vi "XYRange_Default_View.vi"(0 "SygZad Podg Ref":refnum<vi>, 1 "Radio Buttons":T1(radio), 2 "Offset ACDist":dbl, 3 "Offset":dbl, 4 "Amplituda":dbl, 5 "error in (no error)":errorcluster) -> (19 "error out":errorcluster)   [LabVIEW 2021]
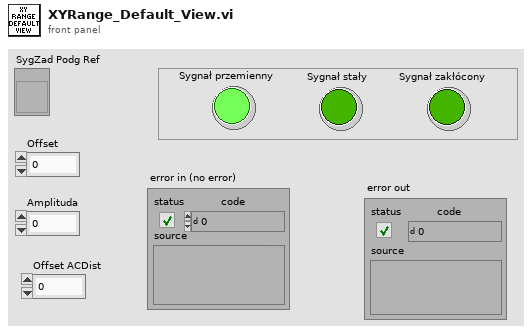
[diagram p1: front panel]
types:
  T1 = enum32{"Sygnał przemienny", "Sygnał stały", "Sygnał zakłócony"}
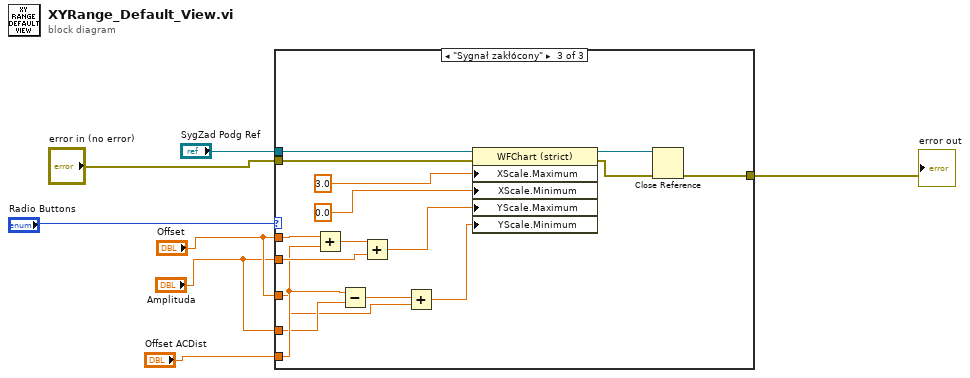
[diagram p0: block diagram]
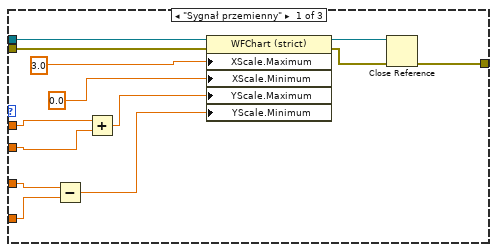
[diagram p2: hidden frame]
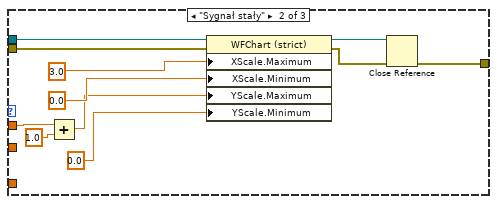
[diagram p3: hidden frame]
diagram:
  n1 = case shown="\"Sygnał zakłócony\"" "Radio Buttons" {
    tunnel: "SygZad Podg Ref" -> [w20 w31 w47]
    tunnel: "error in (no error)" -> [w18 w29 w45]
    tunnel: [w16 w27 w43] -> w5
    tunnel: "Offset" -> [w8 w24 w40]
    tunnel: "Amplituda" -> [w12 _ w38]
    tunnel: "Offset" -> [w11 _ w33]
    tunnel: "Amplituda" -> [w10 _ w35]
    tunnel: "Offset ACDist" -> [_ _ w36]
    frame "Sygnał przemienny" {
      n2 = Subtract(x=w11, y=w10) -> (x-y=w9:dbl)
      n3 = Add(x=w8, y=w12) -> (x+y=w13:dbl)
      n4 = property class="WFChart (strict)"(reference=w20, error in=w18, "XScale.Maximum"=3.0 ("X Scale.Range:Maximum"), "XScale.Minimum"=0.0 ("X Scale.Range:Minimum"), "YScale.Maximum"=w13, "YScale.Minimum"=w9) -> (reference out=w19:refnum<vi>, error out=w17:errorcluster)
      n5 = Close Reference(reference=w19, error in (no error)=w17) -> (error out=w16:errorcluster)
    }
    frame "Sygnał stały" {
      n6 = Add(x=w24, y=1.0) -> (x+y=w23:dbl)
      n7 = property class="WFChart (strict)"(reference=w31, error in=w29, "XScale.Maximum"=3.0 ("X Scale.Range:Maximum"), "XScale.Minimum"=0.0 ("X Scale.Range:Minimum"), "YScale.Maximum"=w23, "YScale.Minimum"=0.0 ("Y Scale.Range:Minimum")) -> (reference out=w30:refnum<vi>, error out=w28:errorcluster)
      n8 = Close Reference(reference=w30, error in (no error)=w28) -> (error out=w27:errorcluster)
    }
    frame "Sygnał zakłócony" {
      n9 = Add(x=w40, y=w36) -> (x+y=w39:dbl)
      n10 = Subtract(x=w36, y=w35) -> (x-y=w34:dbl)
      n11 = Add(x=w39, y=w38) -> (x+y=w37:dbl)
      n12 = Add(x=w34, y=w33) -> (x+y=w32:dbl)
      n13 = property class="WFChart (strict)"(reference=w47, error in=w45, "XScale.Maximum"=3.0 ("X Scale.Range:Maximum"), "XScale.Minimum"=0.0 ("X Scale.Range:Minimum"), "YScale.Maximum"=w37, "YScale.Minimum"=w32) -> (reference out=w46:refnum<vi>, error out=w44:errorcluster)
      n14 = Close Reference(reference=w46, error in (no error)=w44) -> (error out=w43:errorcluster)
    }
  }
  "error out" <- w5
